vi "Invert Histogram.vi"(8 "error in (no error)":errorcluster, 11 "Histogram":cluster{"Axis":dbl[], "Histogram":dbl[]}) -> (0 "error out":errorcluster, 3 "Inverted Histogram":cluster{"Axis":dbl[], "Histogram":dbl[]})   [LabVIEW 2021, in "Histogram Window.lvlib"]
uses:
  Histogram Window.lvlib
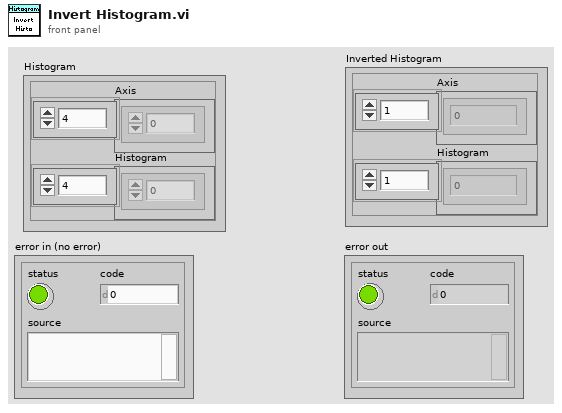
[diagram p1: front panel]
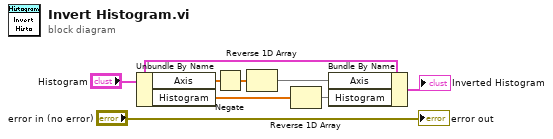
[diagram p0: block diagram]
diagram:
  n1 = Unbundle By Name("Histogram") -> ("Axis"=w5:dbl[], "Histogram"=w3:dbl[])
  n2 = Negate(x=w5) -> (-x=w4:dbl[])
  n3 = Reverse 1D Array(array=w4) -> (reversed array=w1:dbl[])
  n4 = Reverse 1D Array(array=w3) -> (reversed array=w2:dbl[])
  n5 = Bundle By Name(cluster="Histogram", "Axis"=w1, "Histogram"=w2) -> (→"Inverted Histogram":cluster{"Axis":dbl[], "Histogram":dbl[]})
  "error out" <- "error in (no error)"
